vi "GA Get Capture Sense.vi"(8 "error in (no error)":errorcluster caption="错误输入（无错误）", 9 "sense":i16, 10 "mode":i16, 11 "nEncodeNum":i16) -> (0 "error out":errorcluster caption="错误输出", 1 "sense out":i16, 3 "function return":i32)   [LabVIEW 2015, in "GAS.lvlib"]
doc: "extern \"C\" __declspec(dllimport) int GA_GetCaptureSense(short nEncodeNum,short mode,short *sense);"
uses:
  <userlib>/BP_GAS/GAS.lvlib
  <userlib>/BP_GAS/GAS.dll
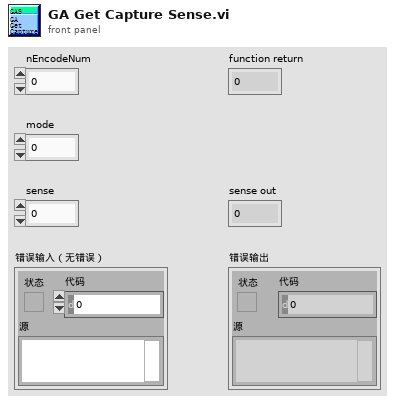
[diagram p1: front panel]
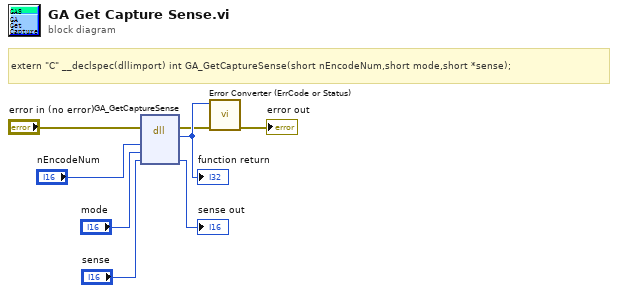
[diagram p0: block diagram]
diagram:
  # "extern \"C\" __declspec(dllimport) int GA_GetCaptureSense(short nEncodeNum,short mode,short *sense);"
  n1 = dll-call lib="E:/Program Files (x86)/National Instruments/LabVIEW 2015/user.lib/BP_GAS/GAS.*" fn="GA_GetCaptureSense"(error in="error in (no error)", "nEncodeNum"="nEncodeNum", "mode"="mode", "sense"="sense") -> (error out=w2:errorcluster, w8:i32, "sense"=→"sense out":i16)  [unwired: 4 in, 1 out]
  "function return" <- w8
  n2 = call "Error Converter (ErrCode or Status).vi"("error in (no error)"=w2, "error code"=w8) -> ("error out"=→"error out":errorcluster)  [unwired: 9 in]
